vi "CheckCom1.vi"(11 "Data In":T2) -> (2 "States":T1=enum."Initialize", 3 "Data Out":T2)   [LabVIEW 2014]
uses:
  controls/Data1.ctl
  controls/Payjson.ctl
  controls/State.ctl
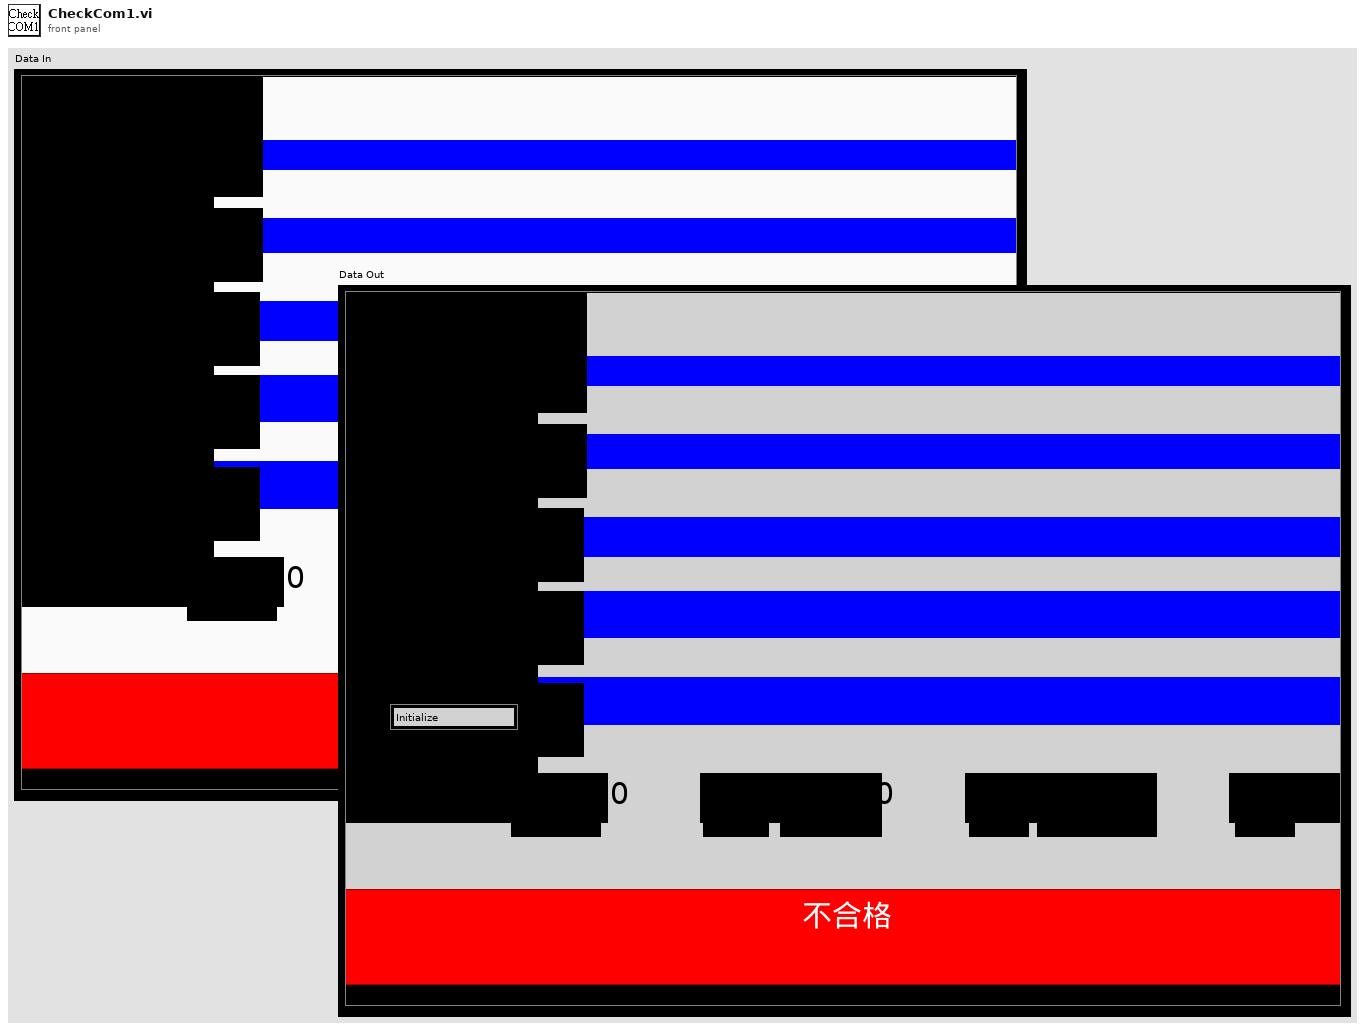
[diagram p1: front panel]
types:
  T1 = typedef "State.ctl" = enum16{"int", "Initalize0", "Initialize", "Wait for Scan", "State 1", "State 2", "NG", "NG1", "OK", "OKNG", "OKNG1", "Exit"}
  T2 = typedef "Data1.ctl" = cluster{"Date":string, "BarCode1":string, "BarCode2":string, "BarCode3":string, "Message":string, "OK Count":u16, "NG Count":u16, "Total Count":u16, "ModelData":string[][], "OK&NG":bool, "COM1":refnum<visa-resource-name>, "COM2":refnum<visa-resource-name>, "IO":i32, "Time":u32, "TCP":refnum<k5>, "TCP 2":refnum<k5>, "COM1 2":refnum<visa-resource-name>, "CheckNum":string, "BarCode1_1":string, "BarCode2_1":string, "BarCode3_1":string, "日期":string, "機種":string, "機號":string, "商品條碼1":string, "OK_1":string, "OK":string, "NG":string, "NG_1":string, "Total":string, "Total_1":string, "ClaerTime":u32, "Pjson":T3, "LotNo":string[], "CheckParsArray":string[], "BarCode4":string, "BarCode4_1":string, "商品條碼2":string, "BarCode5":string, "BarCode5_1":string, "商品條碼3":string, "ReScanNG":i32, "NGTimeCT":u32}
  T3 = typedef "Payjson.ctl" = cluster{"DEPT":string, "LINE":string, "STANO":string, "WORKNO":string, "PRODSN":string, "COMPNTID":string, "COMPNTLOT":string, "COMPNTSN":string, "USEDQTY":i16, "OPDATE":string, "OPUSER":string, "RECVDATE":string, "MMODU":string}[]
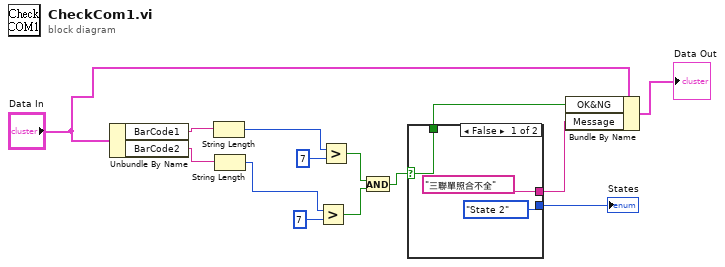
[diagram p0: block diagram]
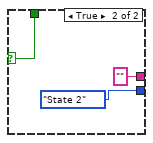
[diagram p2: hidden frame]
diagram:
  n1 = Unbundle By Name("Data In") -> ("BarCode1"=w14:string, "BarCode2"=w11:string)
  n2 = String Length(string=w14) -> (length=w13:i32)
  n3 = String Length(string=w11) -> (length=w10:i32)
  n4 = Greater?(x=w10, y=7) -> (0:w7:bool)
  n5 = Greater?(x=w13, y=7) -> (0:w8:bool)
  n6 = And(x=w8, y=w7) -> (x .and. y?=w6:bool)
  n7 = case shown="False" w6 {
    selector: w6 -> [w17 w20]
    tunnel: [w17 w20] -> w3
    tunnel: ["三聯單照合不全" ""] -> w2
    tunnel: [State."State 2" ("States") State."State 2" ("States")] -> w1
    frame False {
    }
    frame True {
    }
  }
  "States" <- w1
  n8 = Bundle By Name(cluster="Data In", "OK&NG"=w3, "Message"=w2) -> (→"Data Out":T2)
